vi "Get RadioButton Selected Label.vi"(8 "error in (no error)":errorcluster, 11 "Radio Buttons":refnum<vi>) -> (0 "error out":errorcluster, 2 "Label.Text":string, 3 "Radio Buttons out":refnum<vi>)   [LabVIEW 2015]
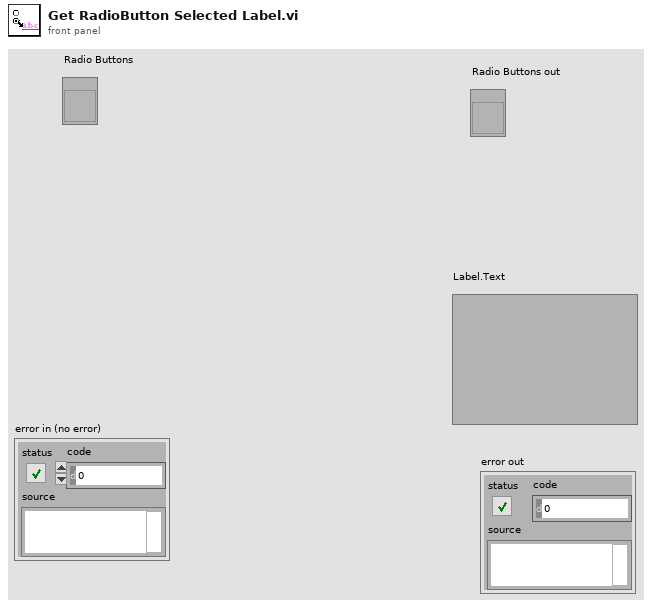
[diagram p1: front panel]
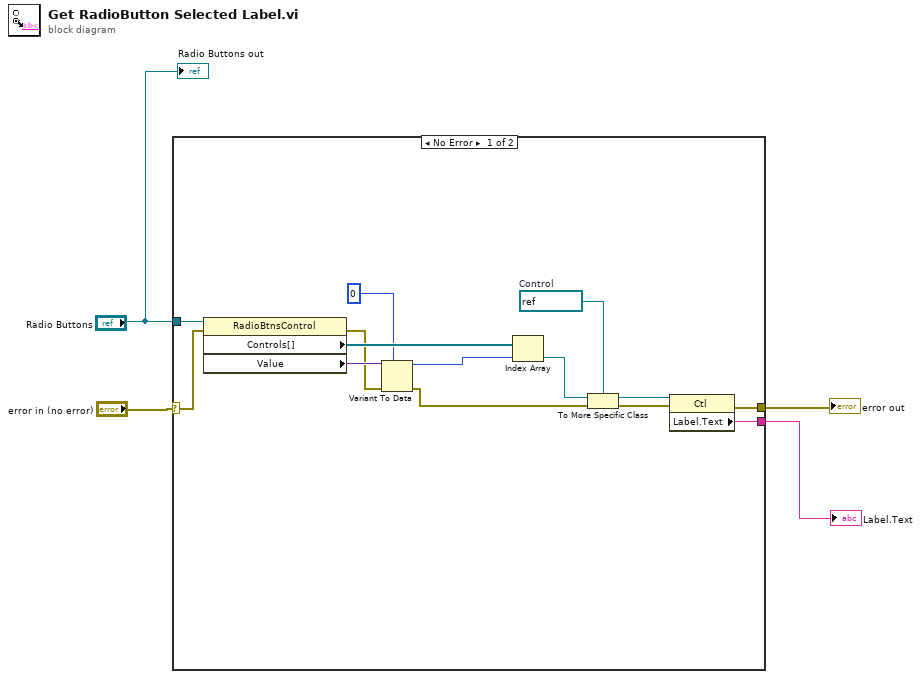
[diagram p0: block diagram]
diagram:
  n1 = case shown="No Error" "error in (no error)" {
    selector: "error in (no error)" -> [w7 w19]
    tunnel: [w6 w19] -> w4
    tunnel: [w5 _] -> w3
    tunnel: "Radio Buttons" -> [w8 _]
    frame No Error {
      w16 = refnum<vi> refnum  # Control
      n2 = property class="RadioBtnsControl"(reference=w8, error in=w7) -> (error out=w10:errorcluster, "Controls[]"=w18:refnum<vi>[], "Value"=w13:variant)  [unwired: 1 out]
      n3 = Variant To Data(error in=w10, type=0 ("index"), Variant=w13) -> (data=w11:i32, error out=w9:errorcluster)
      n4 = Index Array(array=w18, index=w11) -> (element=w17:refnum<vi>)
      n5 = To More Specific Class(target class=w16, reference=w17, error in=w9) -> (specific class reference=w15:refnum<vi>, error out=w14:errorcluster)
      n6 = property on="Property Node" class="Ctl"(reference=w15, error in=w14) -> (error out=w6:errorcluster, "Label.Text"=w5:string)  [unwired: 1 out]
    }
    frame Error {
    }
  }
  "error out" <- w4
  "Label.Text" <- w3
  "Radio Buttons out" <- "Radio Buttons"
